vi "Check for Valid Host Interface.vi"(8 "error in (no error)":errorcluster, 11 "starter kit host in":refnum<class "NI_Robotics_Starter Kit Host_FPGA_1.0.lvclass">) -> (0 "error out":errorcluster, 2 "valid?":bool, 3 "starter kit host out":refnum<class "NI_Robotics_Starter Kit Host_FPGA_1.0.lvclass">)   [LabVIEW 2017, in "NI_Robotics_Starter Kit Host_FPGA_1.0.lvclass"]
uses:
  <vilib>/robotics/Starter Kit/1.0/FPGA Host Interface/NI_Robotics_Starter Kit Host_FPGA_1.0.lvclass
  <vilib>/robotics/Starter Kit/1.0/FPGA Host Interface/NI_Robotics_Starter Kit Host_FPGA_1.0.lvclass/NI_Robotics_Starter Kit Host_FPGA_1.0.ctl
  <vilib>/robotics/Starter Kit/FPGA Host Interface/NI_Robotics_Starter Kit Host_FPGA.lvclass
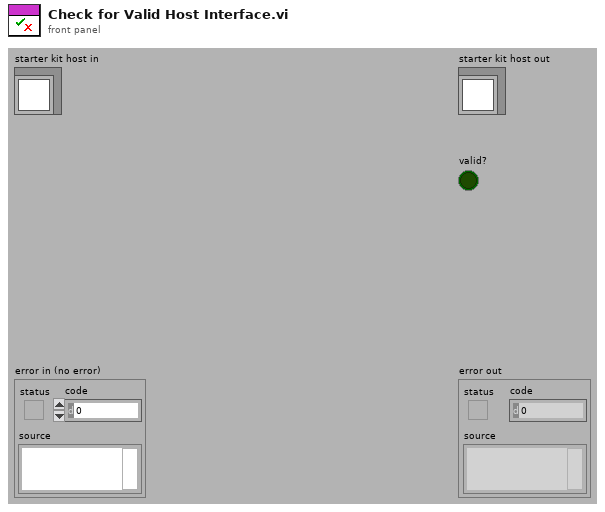
[diagram p1: front panel]
types:
  T1 = typedef "NI_Robotics_Starter Kit Host_FPGA_1.0.lvclass/FPGA Refnum.ctl" = refnum<k20>
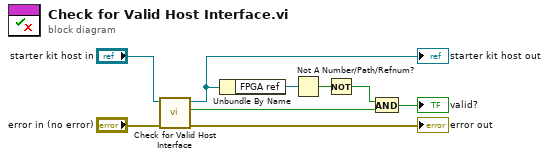
[diagram p0: block diagram]
diagram:
  n1 = call-parent "Check for Valid Host Interface.vi"("error in (no error)"="error in (no error)", "starter kit host in"="starter kit host in") -> ("error out"=→"error out":errorcluster, "valid?"=w3:bool, "starter kit host out"=w4:refnum<class "NI_Robotics_Starter Kit Host_FPGA_1.0.lvclass">)  [unwired: 7 in]
  "starter kit host out" <- w4
  n2 = Unbundle By Name(w4) -> ("FPGA ref"=w9:T1)
  n3 = Not A Number/Path/Refnum?(number/path/refnum=w9) -> (NaN/Path/Refnum?=w8:bool)
  n4 = Not(x=w8) -> (.not. x?=w2:bool)
  n5 = And(x=w2, y=w3) -> (x .and. y?=→"valid?":bool)
